vi "Finish.vi"   [LabVIEW 2015]
doc: "This VI is called just before exiting. It is expected to close I/O refnum, save collected data, etc."
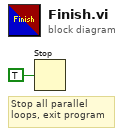
[diagram p0: block diagram]
diagram:
  # "Stop all parallel\nloops, exit program"
  n1 = Stop(stop? (T)=TRUE ("Quit")) -> ()
